vi "FullAdderCircuits.vi"() -> ()   [LabVIEW 2019]
panel:
  out "Carry":bool
  out "SUM":bool
  in  "Input Two":bool
  in  "Input Two":bool
  in  "Input One":bool
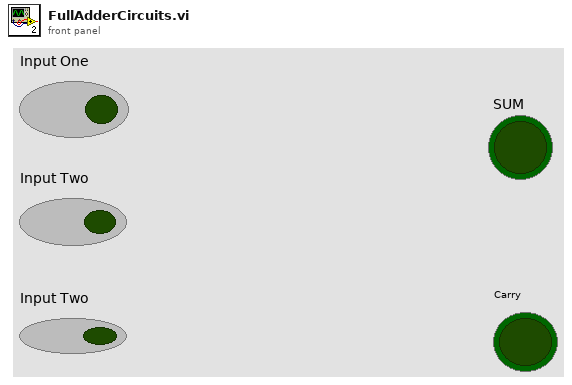
[diagram p1: front panel]
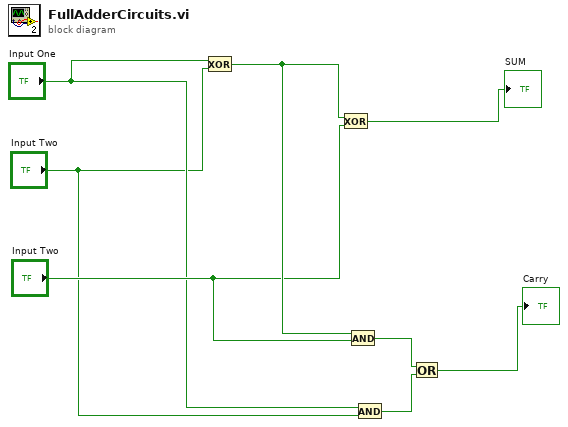
[diagram p0: block diagram]
diagram:
  n1 = Exclusive Or(1:"Input Two", 2:"Input One") -> (0:w7:bool)
  n2 = Exclusive Or(1:"Input Two", 2:w7) -> (0:→"SUM":bool)
  n3 = And(x=w7, y="Input Two") -> (x .and. y?=w3:bool)
  n4 = And(x="Input One", y="Input Two") -> (x .and. y?=w2:bool)
  n5 = Or(x=w3, y=w2) -> (x .or. y?=→"Carry":bool)
